vi "Init Bfr Tx - Data.vi"(7 "Data Access":refnum<class "Data Access Engine.lvclass">, 8 "error in (no error)":errorcluster, 11 "Parameters":variant) -> (0 "error out":errorcluster, 3 "Tx Loop Data":T1={"General Resources"={"Packet Name"="", "Packet ID"=0, "Local IP Address"="", "Local Port"=0, "Multicast"=FALSE, "Multicast IP Address"=0, "Header Info"=[], "Byte Order"=enum."big-endian, network order", "Channel Data Types"=[], "Duplex Packets"=refnum}, "Header Details"={"Packet Size"=0, "Protocol Revision"=0, "System Definition Version"=0, "Source Node Name"="", "Packet ID"=0, "Number of Channels"=0, "Static Header Size"=0, "Total Header Size"=0}, "Buffer Resources"={"Data Buffer"=0, "Pointer Encoding"=enum."Direct Encoding", "Buffer Size"=0, "Buffer Size (I32)"=0, "Raw Buffer Data"=[], "Is Buffered"=FALSE, "External Buffer"=FALSE, "Prepend Header"=FALSE, "Valid Buffer"=FALSE}, "Runtime Resources"={"Connection ID"=refnum, "Transmit Option"=enum."Always", "Destination IP Address"=0, "Destination Port"=0, "Multicast IP Address"=0, "TTL"=0, "Multicast"=FALSE, "Port as Channel"=FALSE, "ExecutionConfig"={"Loop Period"=0, "RT Loop Period"=-2, "Untimed Period"=0, "Target Processor"=0, "Priority"=0, "Thread Management"=enum."Untimed (Default)"}}, "Echo Resources"={"Transmit Echo Option"=enum."PCL Reset", "Packet Count"=0.0, "Counter Increment"=0.0, "Transmit Values"=[]}, "Buffer Option Support"={"Buffer Option"=enum."Static Buffer", "Sim Option"=enum."No Simulation"}, "Channel Resources"={"Transmit Flag"=refnum, "Transmit Echo"=refnum, "Transmit Bytes"=refnum, "Port Channel"=refnum, "Buffer (External)"=refnum, "Buffer (Local)"=refnum, "Timestamp"=refnum}, "Debug Resources"={"Debug Mode"=FALSE, "Debug Log File"=refnum, "Packet Name"=""}} {"Buffer Resources"."Data Buffer" format="%016x"})   [LabVIEW 2019, in "UDP-Custom-Device Engine.lvlib"]
uses:
  UDP-Custom-Device Engine.lvlib
  <vilib>/NI/NIVS Inline Async API/_Data Access Engine/Data Access Engine/Data Access Engine.lvclass
  Types/Engine - Buffered Tx Loop Data.ctl
  Types/Engine - General Resources.ctl
  <vilib>/NI VeriStand/VeriStand Data/Typedefs/Typedefs.Data Types.ctl
  Shared/Types/Shared - Duplex Settings.ctl
  Shared/Types/Shared - Header Details.ctl
  Types/Engine - Buffer Resources.ctl
  Shared/Types/Shared - Pointer Encoding.ctl
  Types/Engine - Tx Runtime Resources.ctl
  Shared/Types/Shared - Transmit Flag Options.ctl
  Types/Engine - Execution Config.ctl
  Shared/Types/Shared - Thread Management.ctl
  Types/Engine - Tx Echo Resources.ctl
  Shared/Types/Shared - Transmit Echo Options.ctl
  Types/Engine - Buffered Tx Buffer Option Support.ctl
  Shared/Types/Shared - Transmit Buffer Options.ctl
  Shared/Types/Shared - Transmit Sim Options.ctl
  Types/Engine - Buffered Tx Channel Refs.ctl
  <vilib>/NI/NIVS Inline Async API/_Data Access Engine/Data Access Engine/Types/Read.DVR.ctl
  <vilib>/NI/NIVS Inline Async API/_Data Access Engine/Access Type Classes/Read/Read.lvclass
  <vilib>/NI/NIVS Inline Async API/_Data Access Engine/Data Access Engine/Types/Write.DVR.ctl
  <vilib>/NI/NIVS Inline Async API/_Data Access Engine/Access Type Classes/Write/Write.lvclass
  Types/Engine - Debug Resources.ctl
  Shared/Types/Shared - Tx.PacketInfo.ctl
  Shared/Types/Shared - Channel Data Type.ctl
  Shared/Types/Shared - Buffered.PacketInfo.ctl
  Shared/Types/Shared - Receive Buffer Options.ctl
  <vilib>/NI/NIVS Inline Async API/_Data Access Engine/Data Access Engine/Methods/Read.Lookup.vi
  <vilib>/NI/NIVS Inline Async API/_Data Access Engine/Data Access Engine/Methods/Write.Lookup.vi
  Shared/UDP-Custom-Device Shared.lvlib
  <vilib>/NI VeriStand/VeriStand Data/VeriStand Data.lvlib
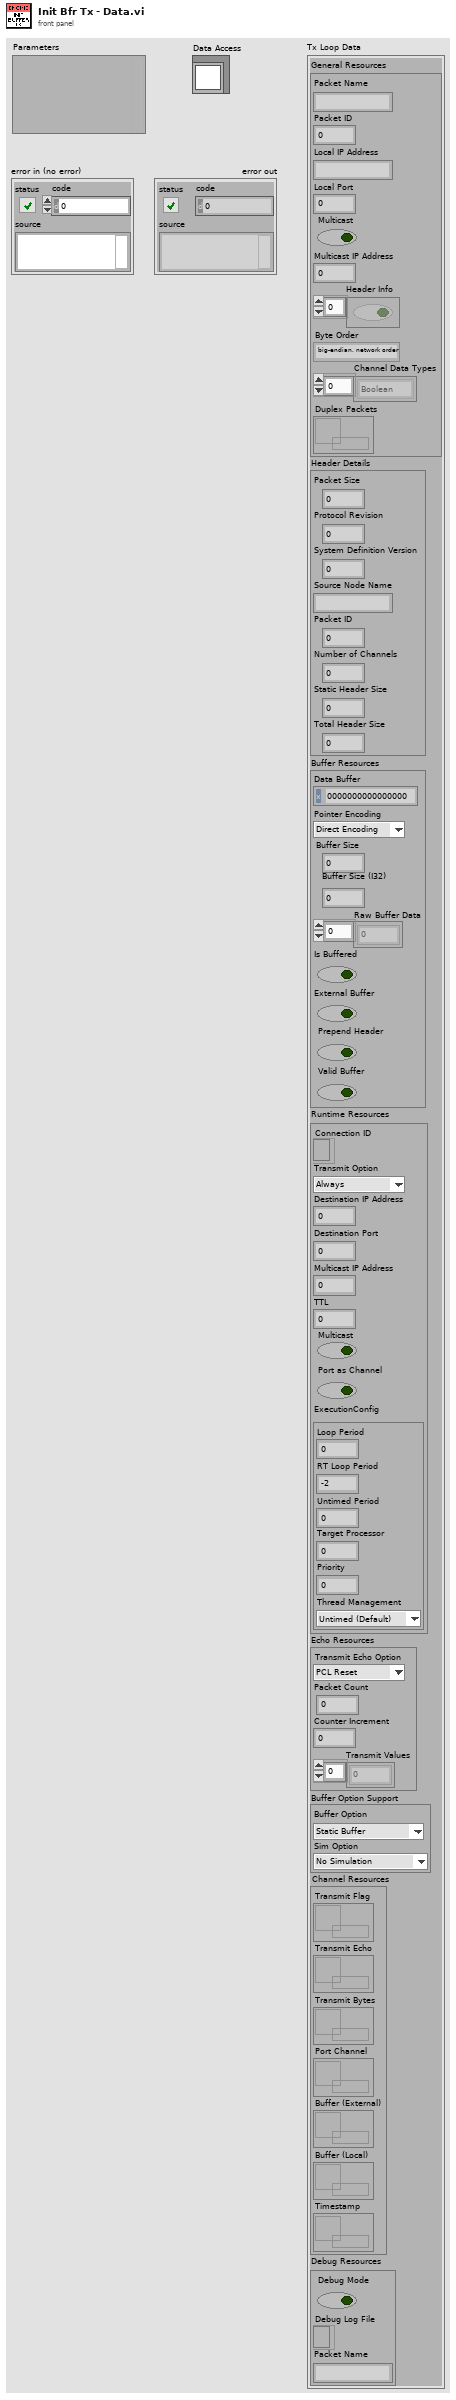
[diagram p1: front panel]
types:
  T1 = typedef "UDP-Custom-Device Engine.lvlib/Engine - Buffered Tx Loop Data.ctl" = cluster{"General Resources":T2, "Header Details":T4, "Buffer Resources":T5, "Runtime Resources":T7, "Echo Resources":T11, "Buffer Option Support":T13, "Channel Resources":T16, "Debug Resources":T19}
  T2 = typedef "UDP-Custom-Device Engine.lvlib/Engine - General Resources.ctl" = cluster{"Packet Name":string, "Packet ID":i32, "Local IP Address":string, "Local Port":i32, "Multicast":bool, "Multicast IP Address":u32, "Header Info":bool[], "Byte Order":enum16{"big-endian, network order", "native, host order", "little-endian"}, "Channel Data Types":T3[], "Duplex Packets":refnum<data-value>}
  T3 = typedef "VeriStand Data.lvlib/Typedefs.Data Types.ctl" = enum16{"Boolean", "Single", "Double", "I8", "I16", "I32", "I64", "U8", "U16", "U32", "U64"}
  T4 = typedef "UDP-Custom-Device Shared.lvlib/Shared - Header Details.ctl" = cluster{"Packet Size":u16, "Protocol Revision":u8, "System Definition Version":u64, "Source Node Name":string, "Packet ID":u32, "Number of Channels":u32, "Static Header Size":u16, "Total Header Size":u16}
  T5 = typedef "UDP-Custom-Device Engine.lvlib/Engine - Buffer Resources.ctl" = cluster{"Data Buffer":u64, "Pointer Encoding":T6, "Buffer Size":u64, "Buffer Size (I32)":i32, "Raw Buffer Data":u8[], "Is Buffered":bool, "External Buffer":bool, "Prepend Header":bool, "Valid Buffer":bool}
  T6 = typedef "UDP-Custom-Device Shared.lvlib/Shared - Pointer Encoding.ctl" = enum16{"Direct Encoding", "Conversion Encoding"}
  T7 = typedef "UDP-Custom-Device Engine.lvlib/Engine - Tx Runtime Resources.ctl" = cluster{"Connection ID":refnum<k16>, "Transmit Option":T8, "Destination IP Address":u32, "Destination Port":u16, "Multicast IP Address":u32, "TTL":u16, "Multicast":bool, "Port as Channel":bool, "ExecutionConfig":T9}
  T8 = typedef "UDP-Custom-Device Shared.lvlib/Shared - Transmit Flag Options.ctl" = enum16{"Always", "One-Shot", "Toggle"}
  T9 = typedef "UDP-Custom-Device Engine.lvlib/Engine - Execution Config.ctl" = cluster{"Loop Period":i64, "RT Loop Period":i64, "Untimed Period":u32, "Target Processor":i32, "Priority":i32, "Thread Management":T10}
  T10 = typedef "UDP-Custom-Device Shared.lvlib/Shared - Thread Management.ctl" = enum16{"Untimed (Default)", "Timed (High Priority)"}
  T11 = typedef "UDP-Custom-Device Engine.lvlib/Engine - Tx Echo Resources.ctl" = cluster{"Transmit Echo Option":T12, "Packet Count":dbl, "Counter Increment":dbl, "Transmit Values":dbl[]}
  T12 = typedef "UDP-Custom-Device Shared.lvlib/Shared - Transmit Echo Options.ctl" = enum16{"PCL Reset", "Counter", "Mirror"}
  T13 = typedef "UDP-Custom-Device Engine.lvlib/Engine - Buffered Tx Buffer Option Support.ctl" = cluster{"Buffer Option":T14, "Sim Option":T15}
  T14 = typedef "UDP-Custom-Device Shared.lvlib/Shared - Transmit Buffer Options.ctl" = enum16{"Static Buffer", "FIFO Buffer", "FIFO Buffer + Port"}
  T15 = typedef "UDP-Custom-Device Shared.lvlib/Shared - Transmit Sim Options.ctl" = enum16{"No Simulation", "Counter", "Full Buffer", "FIFO Test", "FIFO + Port Test"}
  T16 = typedef "UDP-Custom-Device Engine.lvlib/Engine - Buffered Tx Channel Refs.ctl" = cluster{"Transmit Flag":T17, "Transmit Echo":T18, "Transmit Bytes":T17, "Port Channel":T17, "Buffer (External)":T17, "Buffer (Local)":T18, "Timestamp":T17}
  T17 = typedef "Data Access Engine.lvlib/Data Access Engine.lvclass/Read.DVR.ctl" = refnum<data-value>
  T18 = typedef "Data Access Engine.lvlib/Data Access Engine.lvclass/Write.DVR.ctl" = refnum<data-value>
  T19 = typedef "UDP-Custom-Device Engine.lvlib/Engine - Debug Resources.ctl" = cluster{"Debug Mode":bool, "Debug Log File":refnum<file>, "Packet Name":string}
  T20 = typedef "UDP-Custom-Device Shared.lvlib/Shared - Tx.PacketInfo.ctl" = cluster{"Packet Name":string, "Packet ID":i32, "Decimation":u16, "Destination IP Address":string, "Destination Port":u16, "Local IP Address":string, "Local Port":u16, "Endianness":u16, "TTL":u16, "Multicast":bool, "Multicast IP Address":string, "Transmit Option":T8, "Transmit Echo Option":T12, "Transmit Sim Option":T15, "Port as Channel":bool, "Debug Mode":bool, "Header Info":bool[], "Loop Period":u32, "Channel Data Types":T21[], "Header Details":T4, "Buffered Packet Info":T22, "Duplex Packets":refnum<data-value>, "targetProcessor":i8, "targetPriority":i16, "Thread Management":T10}
  T21 = typedef "UDP-Custom-Device Shared.lvlib/Shared - Channel Data Type.ctl" = enum16{"Boolean", "Single", "Double", "I8", "I16", "I32", "I64", "U8", "U16", "U32", "U64"}
  T22 = typedef "UDP-Custom-Device Shared.lvlib/Shared - Buffered.PacketInfo.ctl" = cluster{"Buffer Size":i32, "External Buffer":bool, "Prepend Header":bool, "Is Buffered":bool, "Pointer Encoding":T6, "Rx Buffer Option":T23, "Tx Buffer Option":T14}
  T23 = typedef "UDP-Custom-Device Shared.lvlib/Shared - Receive Buffer Options.ctl" = enum16{"Static Buffer", "Circular Buffer", "Circular Buffer + Size", "Internal Cache", "Internal Cache + Size", "Ping Pong", "Ping Pong + Size"}
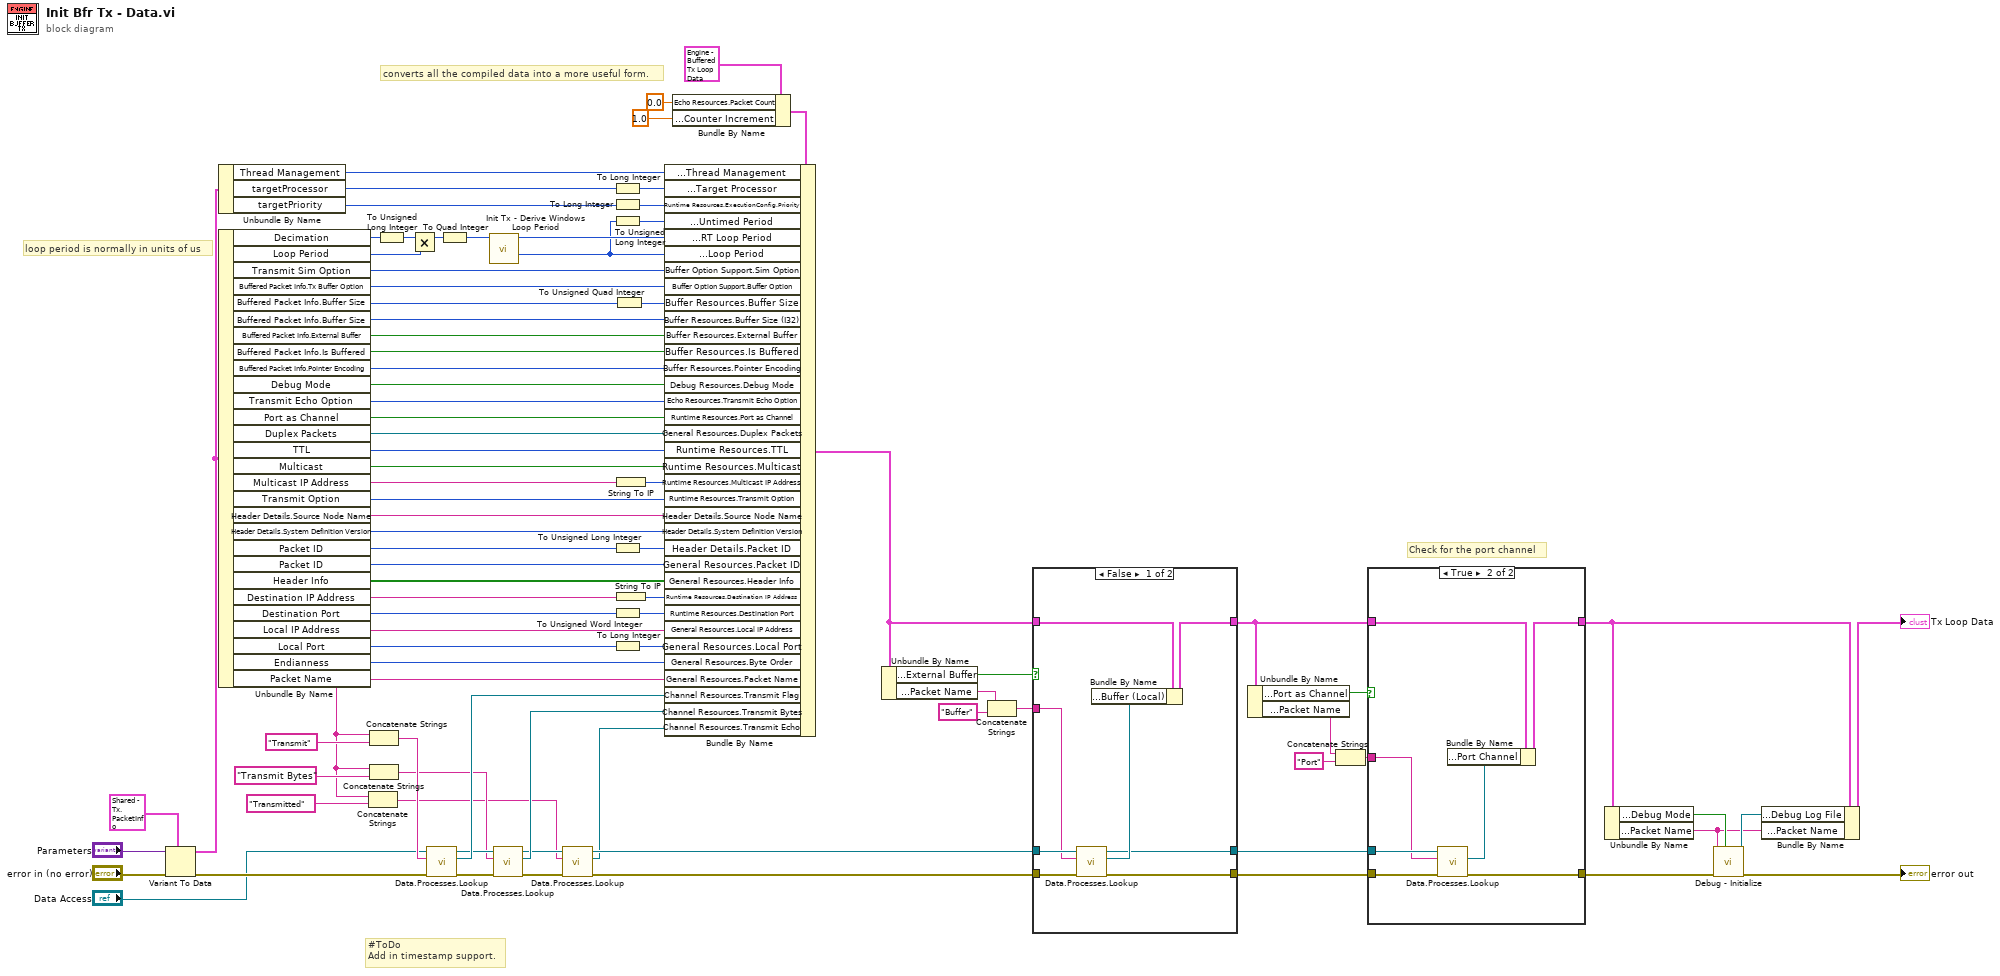
[diagram p0: block diagram]
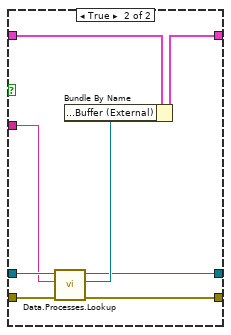
[diagram p3: hidden frame]
diagram:
  # "loop period is normally in units of us"
  # "Check for the port channel"
  # "converts all the compiled data into a more useful form."
  # "#ToDo\nAdd in timestamp support."
  n1 = Variant To Data(error in="error in (no error)", type=T20 {"Packet Name"="", "Packet ID"=0, "Decimation"=0, "Destination IP Address"="", "Destination Port"=0, "Local IP Address"="", "Local Port"=0, "Endianness"=0, "TTL"=0, "Multicast"=FALSE, "Multicast IP Address"="", "Transmit Option"=enum."Always", "Transmit Echo Option"=enum."PCL Reset", "Transmit Sim Option"=enum."No Simulation", "Port as Channel"=FALSE, "Debug Mode"=FALSE, "Header Info"=[], "Loop Period"=0, "Channel Data Types"=[], "Header Details"={"Packet Size"=0, "Protocol Revision"=0, "System Definition Version"=0, "Source Node Name"="", "Packet ID"=0, "Number of Channels"=0, "Static Header Size"=0, "Total Header Size"=0}, "Buffered Packet Info"={"Buffer Size"=0, "External Buffer"=FALSE, "Prepend Header"=FALSE, "Is Buffered"=FALSE, "Pointer Encoding"=enum."Direct Encoding", "Rx Buffer Option"=enum."Static Buffer", "Tx Buffer Option"=enum."Static Buffer"}, "Duplex Packets"=refnum, "targetProcessor"=0, "targetPriority"=1, "Thread Management"=enum."Untimed (Default)"} ("Packet Info"), Variant="Parameters") -> (data=w8:T20, error out=w73:errorcluster)
  n2 = Unbundle By Name(w8) -> ("Thread Management"=w7:T10, "targetProcessor"=w6:i8, "targetPriority"=w5:i16)
  n3 = Unbundle By Name(w8) -> ("Decimation"=w16:u16, "Loop Period"=w15:u32, "Transmit Sim Option"=w19:T15, "Buffered Packet Info.Tx Buffer Option"=w21:T14, "Buffered Packet Info.Buffer Size"=w25:i32, "Buffered Packet Info.Buffer Size"=w1:i32, "Buffered Packet Info.External Buffer"=w26:bool, "Buffered Packet Info.Is Buffered"=w27:bool, "Buffered Packet Info.Pointer Encoding"=w28:T6, "Debug Mode"=w36:bool, "Transmit Echo Option"=w37:T12, "Port as Channel"=w49:bool, "Duplex Packets"=w54:refnum<data-value>, "TTL"=w60:u16, "Multicast"=w61:bool, "Multicast IP Address"=w63:string, "Transmit Option"=w64:T8, "Header Details.Source Node Name"=w86:string, "Header Details.System Definition Version"=w85:u64, "Packet ID"=w14:i32, "Packet ID"=w13:i32, "Header Info"=w83:bool[], "Destination IP Address"=w66:string, "Destination Port"=w82:u16, "Local IP Address"=w81:string, "Local Port"=w78:u16, "Endianness"=w80:u16, "Packet Name"=w44:string)
  n4 = Concatenate Strings(w44, "Transmitted" ("Item GUID")) -> (w38:string)
  n5 = Concatenate Strings(w44, "Transmit" ("Item GUID")) -> (w74:string)
  n6 = Concatenate Strings(w44, "Transmit Bytes" ("Item GUID")) -> (w56:string)
  n7 = To Unsigned Long Integer(number=w16) -> (unsigned 32bit integer=w17:u32)
  n8 = Multiply(x=w17, y=w15) -> (x*y=w18:u32)
  n9 = call-poly <vilib>:"Data.Processes.Lookup.vi"("error in (no error)"=w73, "Name"=w74, "Data Access API in"="Data Access") -> ("error out"=w58:errorcluster, "Ref"=w65:T17, "Data Access API out"=w59:refnum<class "Data Access Engine.lvclass">)  [unwired: 5 in, 1 out]
  n10 = To Quad Integer(1:w18) -> (0:w12:i64)
  n11 = call "Init Tx - Derive Windows Loop Period.vi"("RT Loop Period in"=w12) -> ("Win Loop Period out"=w3:i64, "RT Loop Period out"=w11:i64)  [unwired: 9 in]
  n12 = call-poly <vilib>:"Data.Processes.Lookup.vi"("error in (no error)"=w58, "Name"=w56, "Data Access API in"=w59) -> ("error out"=w41:errorcluster, "Ref"=w55:T17, "Data Access API out"=w43:refnum<class "Data Access Engine.lvclass">)  [unwired: 5 in, 1 out]
  n13 = call-poly <vilib>:"Data.Processes.Lookup.vi"("error in (no error)"=w41, "Name"=w38, "Data Access API in"=w43) -> ("error out"=w40:errorcluster, "Ref"=w39:T18, "Data Access API out"=w42:refnum<class "Data Access Engine.lvclass">)  [unwired: 5 in, 1 out]
  n14 = To Long Integer(number=w6) -> (32bit integer=w10:i32)
  n15 = To Long Integer(number=w5) -> (32bit integer=w9:i32)
  n16 = To Unsigned Long Integer(number=w3) -> (unsigned 32bit integer=w4:u32)
  n17 = To Unsigned Long Integer(number=w14) -> (unsigned 32bit integer=w84:u32)
  n18 = To Unsigned Word Integer(number=w82) -> (unsigned 16bit integer=w79:u16)
  n19 = To Long Integer(number=w78) -> (32bit integer=w77:i32)
  n20 = To Unsigned Quad Integer(1:w25) -> (0:w2:u64)
  n21 = String To IP(1:w63) -> (0:w62:u32)
  n22 = String To IP(1:w66) -> (0:w67:u32)
  n23 = Bundle By Name(cluster=T1 {"General Resources"={"Packet Name"="", "Packet ID"=0, "Local IP Address"="", "Local Port"=0, "Multicast"=FALSE, "Multicast IP Address"=0, "Header Info"=[], "Byte Order"=enum."big-endian, network order", "Channel Data Types"=[], "Duplex Packets"=refnum}, "Header Details"={"Packet Size"=0, "Protocol Revision"=0, "System Definition Version"=0, "Source Node Name"="", "Packet ID"=0, "Number of Channels"=0, "Static Header Size"=0, "Total Header Size"=0}, "Buffer Resources"={"Data Buffer"=0, "Pointer Encoding"=enum."Direct Encoding", "Buffer Size"=0, "Buffer Size (I32)"=0, "Raw Buffer Data"=[], "Is Buffered"=FALSE, "External Buffer"=FALSE, "Prepend Header"=FALSE, "Valid Buffer"=FALSE}, "Runtime Resources"={"Connection ID"=refnum, "Transmit Option"=enum."Always", "Destination IP Address"=0, "Destination Port"=0, "Multicast IP Address"=0, "TTL"=0, "Multicast"=FALSE, "Port as Channel"=FALSE, "ExecutionConfig"={"Loop Period"=0, "RT Loop Period"=-2, "Untimed Period"=0, "Target Processor"=0, "Priority"=0, "Thread Management"=enum."Untimed (Default)"}}, "Echo Resources"={"Transmit Echo Option"=enum."PCL Reset", "Packet Count"=0.0, "Counter Increment"=0.0, "Transmit Values"=[]}, "Buffer Option Support"={"Buffer Option"=enum."Static Buffer", "Sim Option"=enum."No Simulation"}, "Channel Resources"={"Transmit Flag"=refnum, "Transmit Echo"=refnum, "Transmit Bytes"=refnum, "Port Channel"=refnum, "Buffer (External)"=refnum, "Buffer (Local)"=refnum, "Timestamp"=refnum}, "Debug Resources"={"Debug Mode"=FALSE, "Debug Log File"=refnum, "Packet Name"=""}} ("Tx Loop Data"), "Echo Resources.Packet Count"=0.0, "Echo Resources.Counter Increment"=1.0) -> (w23:T1)
  n24 = Bundle By Name(cluster=w23, "Runtime Resources.ExecutionConfig.Thread Management"=w7, "Runtime Resources.ExecutionConfig.Target Processor"=w10, "Runtime Resources.ExecutionConfig.Priority"=w9, "Runtime Resources.ExecutionConfig.Untimed Period"=w4, "Runtime Resources.ExecutionConfig.RT Loop Period"=w11, "Runtime Resources.ExecutionConfig.Loop Period"=w3, "Buffer Option Support.Sim Option"=w19, "Buffer Option Support.Buffer Option"=w21, "Buffer Resources.Buffer Size"=w2, "Buffer Resources.Buffer Size (I32)"=w1, "Buffer Resources.External Buffer"=w26, "Buffer Resources.Is Buffered"=w27, "Buffer Resources.Pointer Encoding"=w28, "Debug Resources.Debug Mode"=w36, "Echo Resources.Transmit Echo Option"=w37, "Runtime Resources.Port as Channel"=w49, "General Resources.Duplex Packets"=w54, "Runtime Resources.TTL"=w60, "Runtime Resources.Multicast"=w61, "Runtime Resources.Multicast IP Address"=w62, "Runtime Resources.Transmit Option"=w64, "Header Details.Source Node Name"=w86, "Header Details.System Definition Version"=w85, "Header Details.Packet ID"=w84, "General Resources.Packet ID"=w13, "General Resources.Header Info"=w83, "Runtime Resources.Destination IP Address"=w67, "Runtime Resources.Destination Port"=w79, "General Resources.Local IP Address"=w81, "General Resources.Local Port"=w77, "General Resources.Byte Order"=w80, "General Resources.Packet Name"=w44, "Channel Resources.Transmit Flag"=w65, "Channel Resources.Transmit Bytes"=w55, "Channel Resources.Transmit Echo"=w39) -> (w70:T1)
  n25 = Unbundle By Name(w70) -> ("Buffer Resources.External Buffer"=w71:bool, "General Resources.Packet Name"=w69:string)
  n26 = Concatenate Strings(w69, "Buffer" ("Item GUID")) -> (w68:string)
  n27 = case shown="False" w71 {
    tunnel: [w93 w101] -> w52
    tunnel: w70 -> [w94 w102]
    tunnel: [w91 w99] -> w51
    tunnel: w40 -> [w92 w100]
    tunnel: w42 -> [w97 w105]
    tunnel: w68 -> [w96 w104]
    tunnel: [w90 w98] -> w50
    frame False {
      n28 = call-poly <vilib>:"Data.Processes.Lookup.vi"("error in (no error)"=w92, "Name"=w96, "Data Access API in"=w97) -> ("error out"=w91:errorcluster, "Ref"=w95:T18, "Data Access API out"=w90:refnum<class "Data Access Engine.lvclass">)  [unwired: 5 in, 1 out]
      n29 = Bundle By Name(cluster=w94, "Channel Resources.Buffer (Local)"=w95) -> (w93:T1)
    }
    frame True {
      n30 = call-poly <vilib>:"Data.Processes.Lookup.vi"("error in (no error)"=w100, "Name"=w104, "Data Access API in"=w105) -> ("error out"=w99:errorcluster, "Ref"=w103:T17, "Data Access API out"=w98:refnum<class "Data Access Engine.lvclass">)  [unwired: 5 in, 1 out]
      n31 = Bundle By Name(cluster=w102, "Channel Resources.Buffer (External)"=w103) -> (w101:T1)
    }
  }
  n32 = Unbundle By Name(w52) -> ("Runtime Resources.Port as Channel"=w53:bool, "General Resources.Packet Name"=w47:string)
  n33 = Concatenate Strings(w47, "Port" ("Item GUID")) -> (w46:string)
  n34 = case shown="True" w53 {
    tunnel: w50 -> [_ w114]
    tunnel: w51 -> [w106 w113]
    tunnel: [w106 w112] -> w34
    tunnel: w52 -> [w107 w111]
    tunnel: [w107 w110] -> w32
    tunnel: w46 -> [_ w109]
    frame False {
    }
    frame True {
      n35 = call-poly <vilib>:"Data.Processes.Lookup.vi"("error in (no error)"=w113, "Name"=w109, "Data Access API in"=w114) -> ("error out"=w112:errorcluster, "Ref"=w108:T17)  [unwired: 5 in, 2 out]
      n36 = Bundle By Name(cluster=w111, "Channel Resources.Port Channel"=w108) -> (w110:T1)
    }
  }
  n37 = Unbundle By Name(w32) -> ("Debug Resources.Debug Mode"=w31:bool, "General Resources.Packet Name"=w29:string)
  n38 = call "Debug - Initialize.vi"("Debug Mode"=w31, "error in (no error)"=w34, "Packet Name"=w29) -> ("error out"=→"error out":errorcluster, "Debug Log File"=w30:refnum<file>)  [unwired: 7 in]
  n39 = Bundle By Name(cluster=w32, "Debug Resources.Debug Log File"=w30, "Debug Resources.Packet Name"=w29) -> (→"Tx Loop Data":T1)
